vi "Traffic_lights-final-random-values.vi"() -> ()   [LabVIEW 2019]
uses:
  <vilib>/numeric/Random Number (Range) U64.vi
  <vilib>/numeric/sub_Random U32.vi
panel:
  out "while index":dbl
  out "horizontal cars sum":dbl
  out "vertical cars sum":dbl
  out "cars vertical 3":dbl
  out "cars vertical 2":dbl
  out "cars horizontal 2":dbl
  out "red 4":bool
  out "green4":bool
  out "red 3":bool
  out "green\n 3":bool
  out "red 2":bool
  out "green\n 2":bool
  out "red":bool
  out "green":bool
  out "cars horizontal":dbl
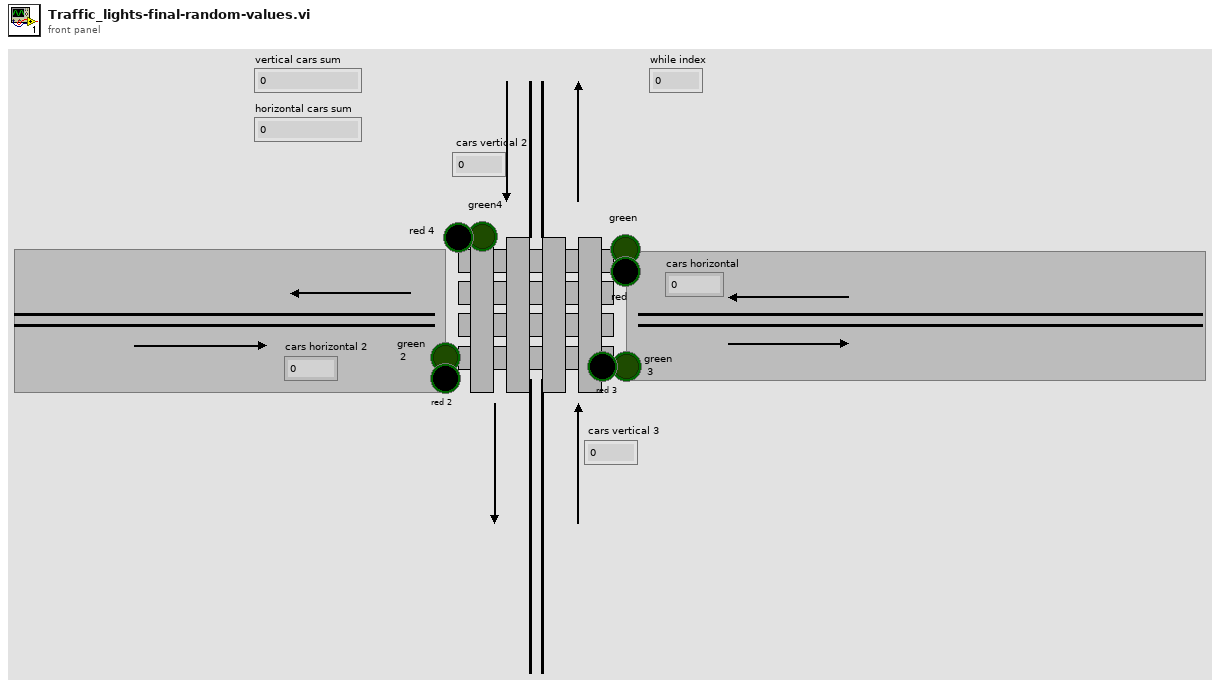
[diagram p1: front panel]
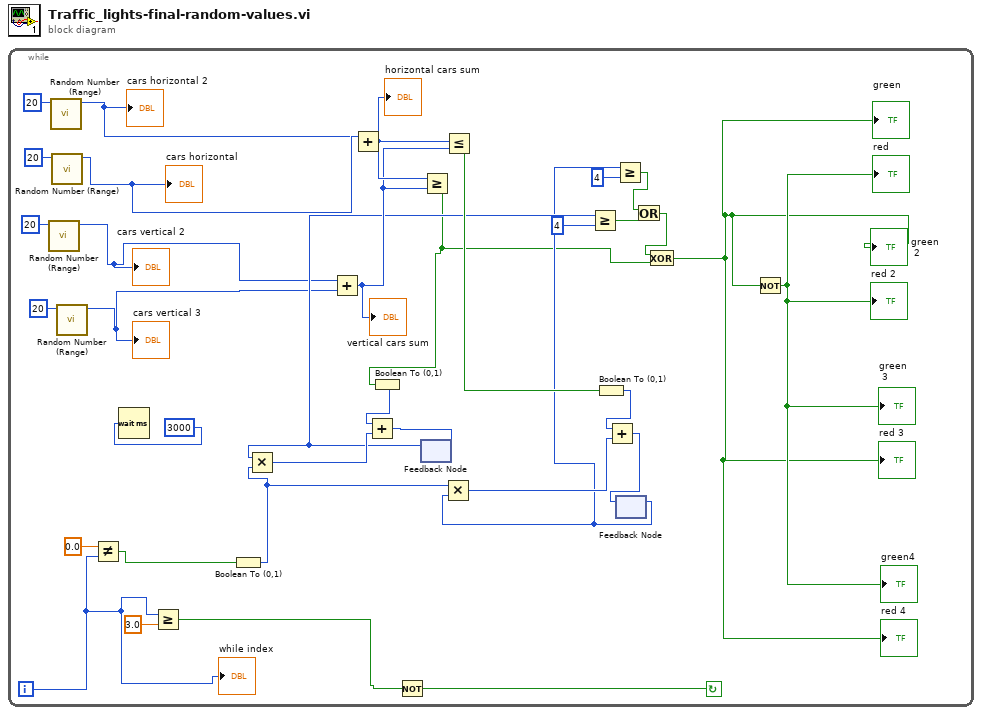
[diagram p0: block diagram]
diagram:
  n1 = while {
    i -> [w15]
    stop <- w30 continue-if-true
    n2 = call-poly <vilib>:"Random Number (Range).vi"("upper bound (100)"=u64 20) -> ("number"=w6:u64)  [unwired: 10 in]
    "cars vertical 2" <- w6
    n3 = call-poly <vilib>:"Random Number (Range).vi"("upper bound (100)"=u64 20) -> ("number"=w7:u64)  [unwired: 10 in]
    "cars horizontal 2" <- w7
    n4 = call-poly <vilib>:"Random Number (Range).vi"("upper bound (100)"=u64 20) -> ("number"=w8:u64)  [unwired: 10 in]
    "cars horizontal" <- w8
    n5 = call-poly <vilib>:"Random Number (Range).vi"("upper bound (100)"=u64 20) -> ("number"=w5:u64)  [unwired: 10 in]
    "cars vertical 3" <- w5
    n6 = Not Equal?(x=0.0, y=w15) -> (x != y?=w14:bool)
    n7 = Wait (ms)(milliseconds to wait=u32 3000) -> ()  [unwired: 1 out]
    n8 = Greater Or Equal?(x=w15, y=3.0) -> (x >= y?=w31:bool)
    n9 = Boolean To (0,1)(Boolean=w14) -> (0, 1=w21:i16)
    n10 = Add(x=w6, y=w5) -> (x+y=w26:u64)
    "vertical cars sum" <- w26
    n11 = Add(x=w8, y=w7) -> (x+y=w27:u64)
    "horizontal cars sum" <- w27
    n12 = Not(x=w31) -> (.not. x?=w30:bool)
    n13 = feedback #1() -> (w13:i16)  [unwired: 1 in]
    n14 = Multiply(x=w13, y=w21) -> (x*y=w29:i16)
    n15 = Greater Or Equal?(x=w27, y=w26) -> (x >= y?=w10:bool)
    n16 = Boolean To (0,1)(Boolean=w10) -> (0, 1=w32:i16)
    n17 = Add(x=w32, y=w29) -> (x+y=w17:i16)
    n18 = feedback-in #1(w17) -> ()
    n19 = Less Or Equal?(x=w27, y=w26) -> (x <= y?=w25:bool)
    n20 = Greater Or Equal?(x=w13, y=i16 4) -> (x >= y?=w19:bool)
    n21 = Boolean To (0,1)(Boolean=w25) -> (0, 1=w24:i16)
    n22 = feedback #2() -> (w12:i16)  [unwired: 1 in]
    n23 = Multiply(x=w21, y=w12) -> (x*y=w20:i16)
    n24 = Add(x=w24, y=w20) -> (x+y=w23:i16)
    n25 = Greater Or Equal?(x=w12, y=i16 4) -> (x >= y?=w18:bool)
    n26 = feedback-in #2(w23) -> ()
    n27 = Or(x=w18, y=w19) -> (x .or. y?=w11:bool)
    n28 = Exclusive Or(1:w10, 2:w11) -> (0:w9:bool)
    "green" <- w9
    "green\n 2" <- w9
    "red 3" <- w9
    "red 4" <- w9
    n29 = Not(x=w9) -> (.not. x?=→"red" →"red 2" →"green\n 3" →"green4":bool)
    "while index" <- w15
  }
